vi "7HP_Create datalog header string - PC.vi"() -> (0 "Datalog header string":string)   [LabVIEW 2021]
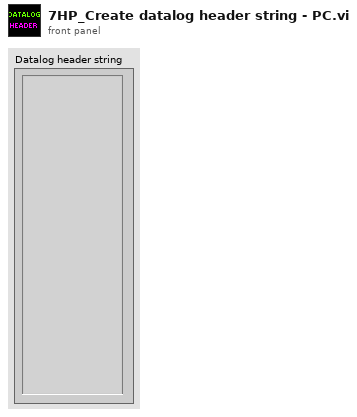
[diagram p1: front panel]
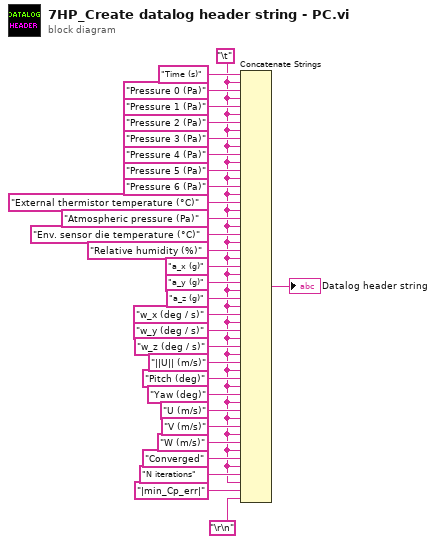
[diagram p0: block diagram]
diagram:
  w3 = "\t"
  n1 = Concatenate Strings("Time (s)", w3, "Pressure 0 (Pa)", w3, "Pressure 1 (Pa)", w3, "Pressure 2 (Pa)", w3, "Pressure 3 (Pa)", w3, "Pressure 4 (Pa)", w3, "Pressure 5 (Pa)", w3, "Pressure 6 (Pa)", w3, "External thermistor temperature (°C)", w3, "Atmospheric pressure (Pa)", w3, "Env. sensor die temperature (°C)", w3, "Relative humidity (%)", w3, "a_x (g)", w3, "a_y (g)", w3, "a_z (g)", w3, "w_x (deg / s)", w3, "w_y (deg / s)", w3, "w_z (deg / s)", w3, "||U|| (m/s)", w3, "Pitch (deg)", w3, "Yaw (deg)", w3, "U (m/s)", w3, "V (m/s)", w3, "W (m/s)", w3, "Converged", w3, "N iterations", w3, "|min_Cp_err|", "\r\n") -> (→"Datalog header string":string)
